vi "Group_Start Wfms.vi"(8 "error in (no error)":errorcluster, 11 "Group in":refnum<class "Group.lvclass">) -> (0 "error out":errorcluster, 3 "Group out":refnum<class "Group.lvclass">)   [LabVIEW 2023, in "Group.lvclass"]
doc: "Starts the waveform sessions on it's subsidary waveform channels."
uses:
  Group.lvclass
  Group.lvclass/Group.ctl
  Channel/Channel.lvclass
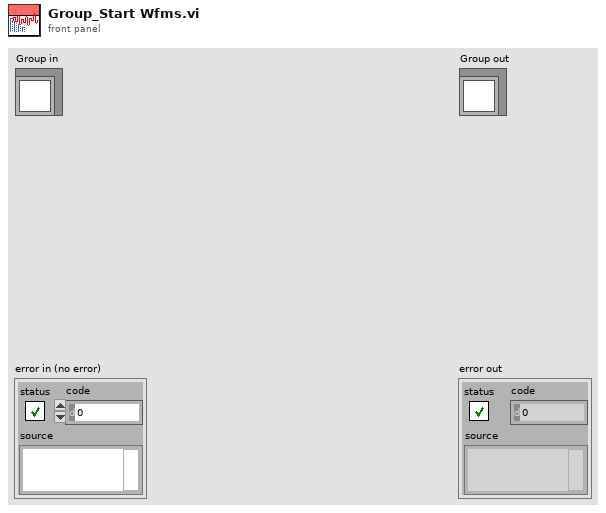
[diagram p1: front panel]
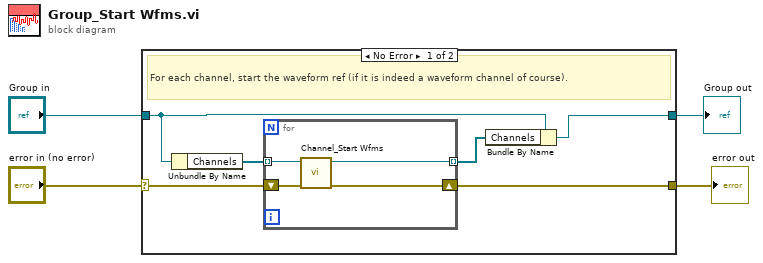
[diagram p0: block diagram]
diagram:
  n1 = case shown="No Error" "error in (no error)" {
    selector: "error in (no error)" -> [w6 w16]
    tunnel: [w5 w16] -> w3
    tunnel: [w9 w15] -> w1
    tunnel: "Group in" -> [w8 w15]
    frame No Error {
      # "For each channel, start the waveform ref (if it is indeed a waveform channel of course)."
      n2 = Unbundle By Name(w8) -> ("Channels"=w10:refnum<class "Channel.lvclass">[])
      n3 = for {
        tunnel: w10 -> [w14] mode=indexing
        tunnel: [w13] -> w7 mode=indexing
        shift-right: [w11] -> w5
        shift-left: w6 -> [w12]
        n4 = call-dynamic "Channel_Start Wfms.vi"("error in (no error)"=w12, "Channel in"=w14) -> ("error out"=w11:errorcluster, "Channel out"=w13:refnum<class "Channel.lvclass">)  [unwired: 8 in]
      }
      n5 = Bundle By Name(cluster=w8, "Channels"=w7) -> (w9:refnum<class "Group.lvclass">)
    }
    frame Error {
    }
  }
  "error out" <- w3
  "Group out" <- w1
